vi "Vision Processing.vi"(4 "error in (no error)":errorcluster, 7 "Image Size":T1=enum."320x240") -> ()   [LabVIEW 2019]
doc: "This VI runs in parallel to other tasks. It gets images from the camera, processes them for color or shape and use that information to affect robot behavior."
uses:
  <vilib>/Rock Robotics/WPI/Camera/WPI_CameraImageSize.ctl
  <vilib>/Rock Robotics/WPI/Camera/WPI_CameraWhite Balance Values.ctl
  <vilib>/Rock Robotics/WPI/Camera/WPI_CameraExposure Values.ctl
  <vilib>/Rock Robotics/WPI/Camera/WPI_CameraFrameRate.ctl
  Robot Global Data.vi
  <vilib>/Rock Robotics/Network Tables/NT Write Number.vi
  <vilib>/Rock Robotics/Network Tables/NT Write Boolean.vi
  <vilib>/vision/driver/NI_Vision_Acquisition_Software.lvlib
  <vilib>/userDefined/High Color/IMAQdx.ctl
panel:
  out "x = y?":bool
  in  "Distance 2":u32
  out "f 2":dbl
  out "Object Size 2":u32
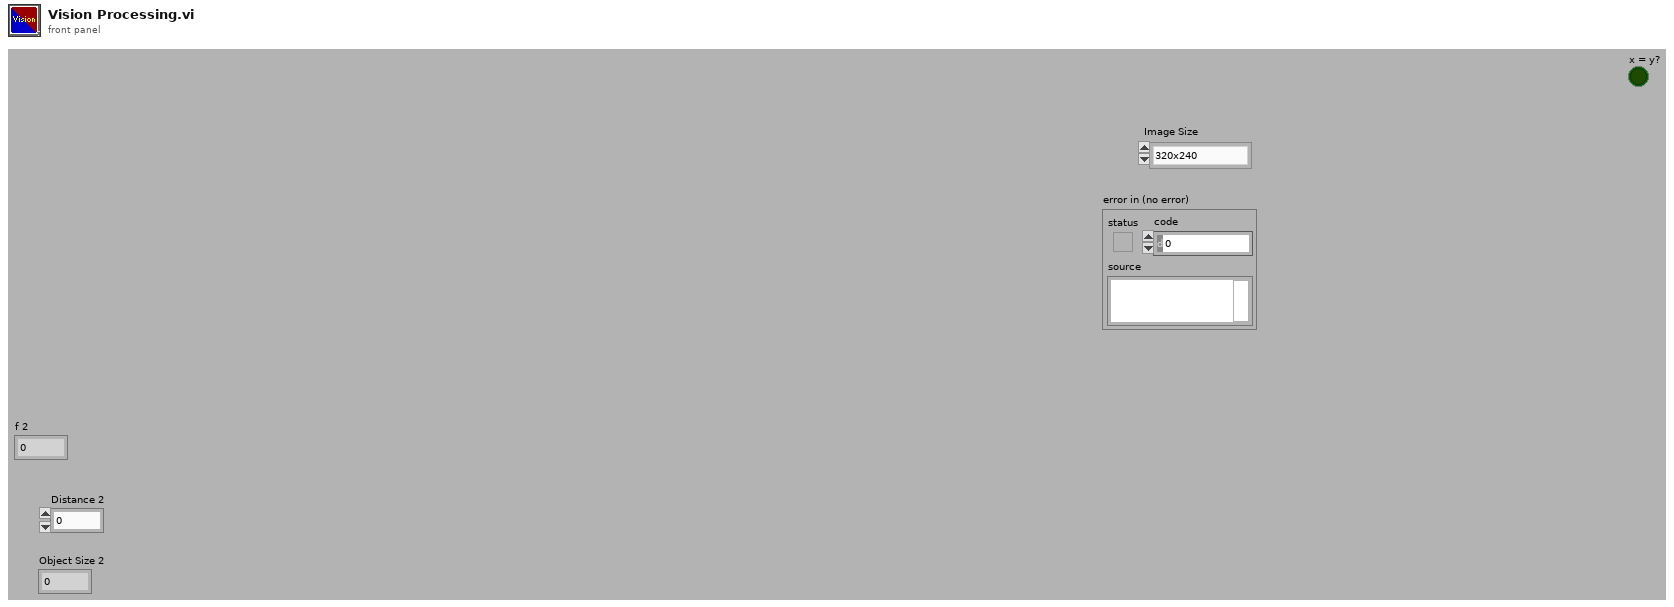
[diagram p1: front panel]
types:
  T1 = typedef "WPI_CameraImageSize.ctl" = enum16{"640x480", "320x240", "160x120", "Custom"}
  T2 = typedef "WPI_MotorControlDeviceRef.ctl" = cluster{"DeviceStatus":errorcluster, "Type":T3, "PWM":cluster{"PWM Channel":T4, "DeadBand":T5}, "CAN":cluster{"Device Number":u8, "SetOutput VI Ref":variant, "GetOutput VI Ref":variant, "Enable VI Ref":variant, "Disable VI Ref":variant, "Data":variant}, "Invert":bool, "DIO PWM":cluster{"PWM \"Enable\" Channel":T4, "DIOChannel":T6, "PWM Rate":dbl}}
  T3 = typedef "WPI_MotorControlType.ctl" = enum16{"PWM", "CAN", "DIO PWM"}
  T4 = typedef "FPGA_DIOPWMChannel.ctl" = enum8{"PWM 0", "PWM 1", "PWM 2", "PWM 3", "PWM 4", "PWM 5", "PWM 6", "PWM 7", "PWM 8", "PWM 9", "PWM MXP 0", "PWM MXP 1", "PWM MXP 2", "PWM MXP 3", "PWM MXP 4", "PWM MXP 5", "PWM MXP 6", "PWM MXP 7", "PWM MXP 8", "PWM MXP 9", "Invalid"}
  T5 = typedef "WPI_PWMDeadband.ctl" = cluster{"Name":string, "maxPositivePwm":i32, "minPositivePwm":i32, "centerPwm":i32, "maxNegativePwm":i32, "minNegativePwm":i32, "angularRange":u16}
  T6 = typedef "FPGA_DIOChannel.ctl" = enum8{"DIO 0", "DIO 1", "DIO 2", "DIO 3", "DIO 4", "DIO 5", "DIO 6", "DIO 7", "DIO 8", "DIO 9", "DIO MXP 0", "DIO MXP 1", "DIO MXP 2", "DIO MXP 3", "DIO MXP 4", "DIO MXP 5", "DIO MXP 6", "DIO MXP 7", "DIO MXP 8", "DIO MXP 9", "DIO MXP 10", "DIO MXP 11", "DIO MXP 12", "DIO MXP 13", "DIO MXP 14", "DIO MXP 15", "SPI Port CS1", "SPI Port CS2", "SPI Port CS3", "SPI Port MISO", "SPI Port MOSI", "Invalid"}
  T7 = typedef "WPI_CameraFrameRate.ctl" = u32
  T8 = typedef "WPI_CameraExposure Values.ctl" = enum16{"Auto", "Flicker-free 50 Hz", "Flicker-free 60 Hz", "Hold current", "Custom"}
  T9 = typedef "WPI_CameraWhite Balance Values.ctl" = enum16{"Auto", "Fixed indoor", "Fixed outdoor 1", "Fixed outdoor 2", "Fixed fluorescent 1", "Fixed fluorescent 2", "Hold current", "Custom"}
  T10 = typedef "IMAQdx.ctl" = refnum<k21>
  T11 = typedef "Image Type" = u32
  T12 = typedef "WPI_CameraDevRef.ctl" = cluster{"Camera Address":string, "CameraStatus":errorcluster}
  T13 = typedef "IMAQ Image.ctl" = refnum<image>
  T14 = cluster{"Global Rectangle":cluster{"x1Left":i32, "y1Top":i32, "x2Right":i32, "y2Bottom":i32}, "Centroid":cluster{"x":sgl, "y":sgl}, "Object Size":u32, "Score":dbl}[]
  T15 = cluster{"Global Rectangle":cluster{"x1Left":i32, "y1Top":i32, "x2Right":i32, "y2Bottom":i32}, "Centroid":cluster{"x":sgl, "y":sgl}, "Object Size":u32, "Score":dbl}
  T16 = cluster{"Shape Report[0]":cluster{"Global Rectangle":cluster{"x1Left":i32, "y1Top":i32, "x2Right":i32, "y2Bottom":i32}, "Centroid":cluster{"x":sgl, "y":sgl}, "Object Size":u32, "Score":dbl}, "Shape Report[1]":cluster{"Global Rectangle":cluster{"x1Left":i32, "y1Top":i32, "x2Right":i32, "y2Bottom":i32}, "Centroid":cluster{"x":sgl, "y":sgl}, "Object Size":u32, "Score":dbl}, "Shape Report[2]":cluster{"Global Rectangle":cluster{"x1Left":i32, "y1Top":i32, "x2Right":i32, "y2Bottom":i32}, "Centroid":cluster{"x":sgl, "y":sgl}, "Object Size":u32, "Score":dbl}, "Shape Report[3]":cluster{"Global Rectangle":cluster{"x1Left":i32, "y1Top":i32, "x2Right":i32, "y2Bottom":i32}, "Centroid":cluster{"x":sgl, "y":sgl}, "Object Size":u32, "Score":dbl}, "Shape Report[4]":cluster{"Global Rectangle":cluster{"x1Left":i32, "y1Top":i32, "x2Right":i32, "y2Bottom":i32}, "Centroid":cluster{"x":sgl, "y":sgl}, "Object Size":u32, "Score":dbl}, "Shape Report[5]":cluster{"Global Rectangle":cluster{"x1Left":i32, "y1Top":i32, "x2Right":i32, "y2Bottom":i32}, "Centroid":cluster{"x":sgl, "y":sgl}, "Object Size":u32, "Score":dbl}, "Shape Report[6]":cluster{"Global Rectangle":cluster{"x1Left":i32, "y1Top":i32, "x2Right":i32, "y2Bottom":i32}, "Centroid":cluster{"x":sgl, "y":sgl}, "Object Size":u32, "Score":dbl}, "Shape Report[7]":cluster{"Global Rectangle":cluster{"x1Left":i32, "y1Top":i32, "x2Right":i32, "y2Bottom":i32}, "Centroid":cluster{"x":sgl, "y":sgl}, "Object Size":u32, "Score":dbl}, "Shape Report[8]":cluster{"Global Rectangle":cluster{"x1Left":i32, "y1Top":i32, "x2Right":i32, "y2Bottom":i32}, "Centroid":cluster{"x":sgl, "y":sgl}, "Object Size":u32, "Score":dbl}}
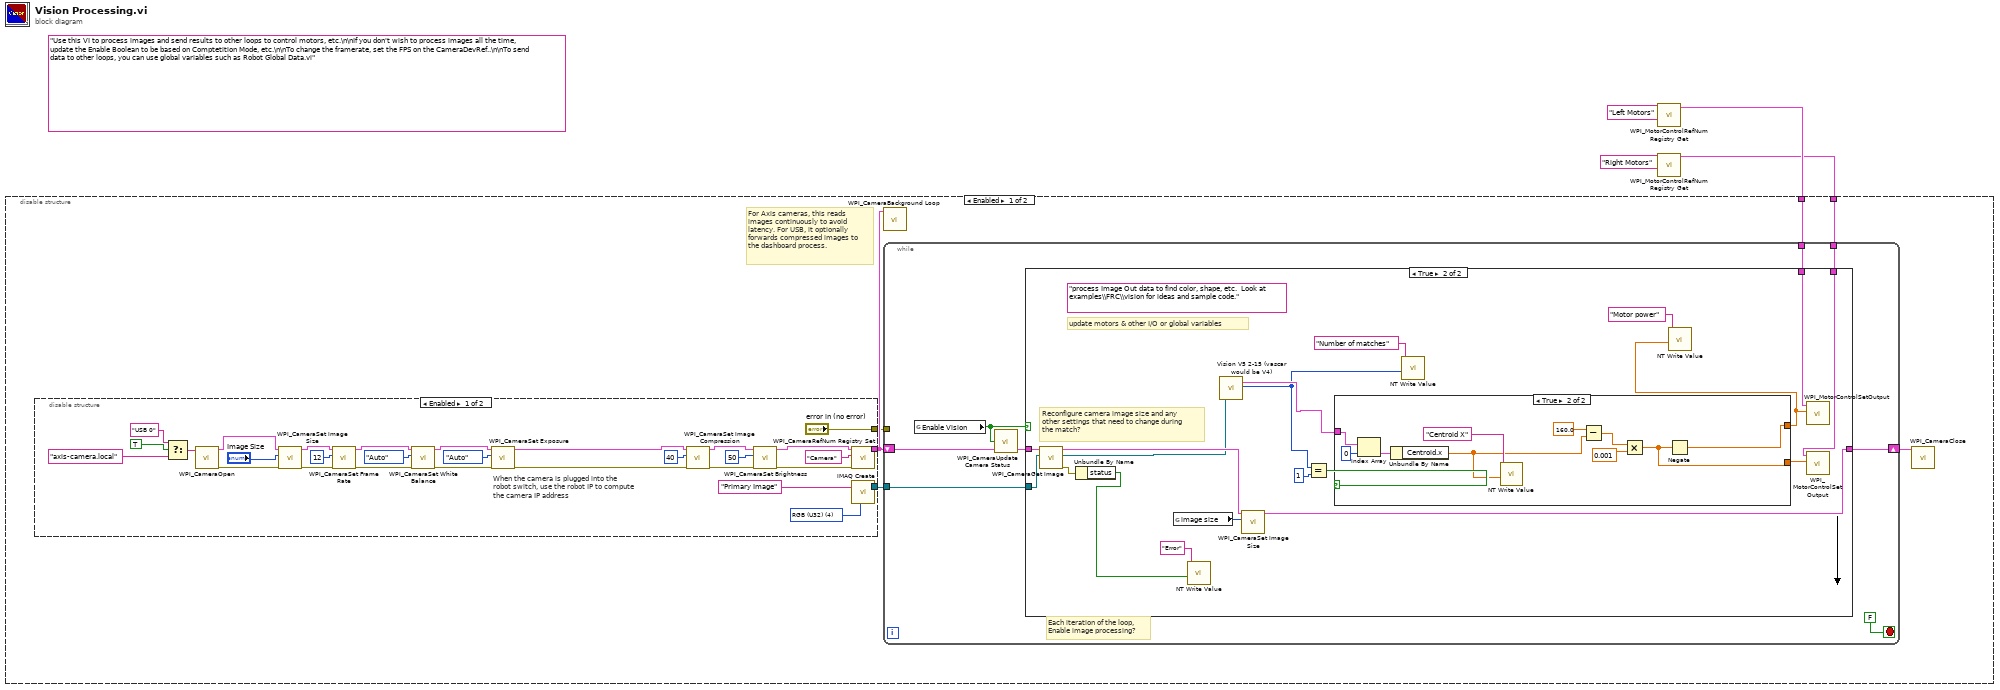
[diagram p0: block diagram]
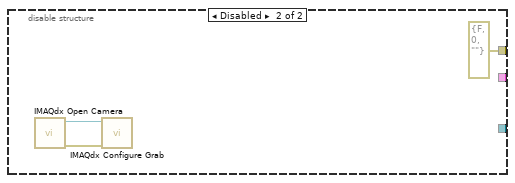
[diagram p2: hidden frame]
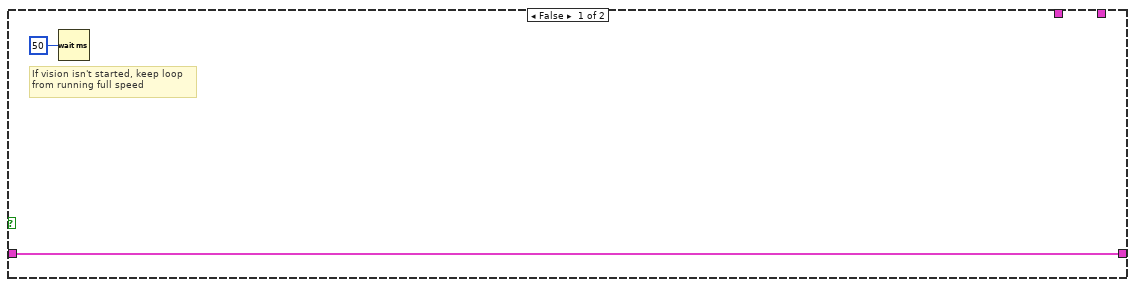
[diagram p3: hidden frame]
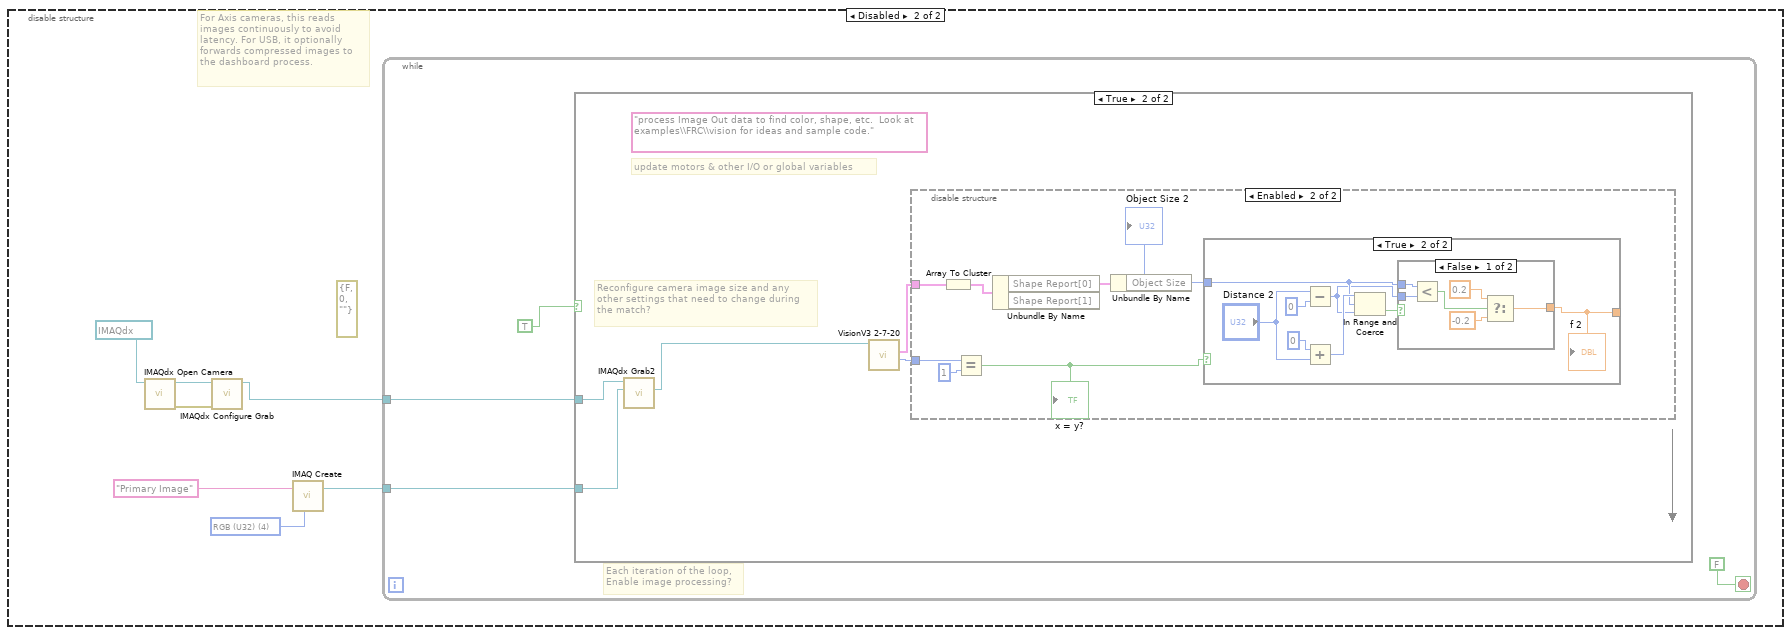
[diagram p5: hidden frame]
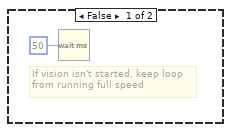
[diagram p6: hidden frame]
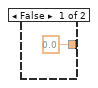
[diagram p8: hidden frame]
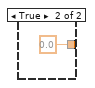
[diagram p9: hidden frame]
diagram:
  (unwired) "Use this VI to process images and send results to other loops to control motors, etc.\n\nIf you don't wish to process images all the time, update the Enable Boolean to be based on Comptetition Mode, etc.\n\nTo change the framerate, set the FPS on the CameraDevRef..\n\nTo send data to other loops, you can use global variables such as Robot Global Data.vi"
  n1 = call <vilib>:"WPI_MotorControlRefNum Registry Get.vi"("refnum name"="Left Motors") -> ("MotorControlDevRef"=w4:T2)  [unwired: 9 in, 1 out]
  n2 = call <vilib>:"WPI_MotorControlRefNum Registry Get.vi"("refnum name"="Right Motors") -> ("MotorControlDevRef"=w3:T2)  [unwired: 9 in, 1 out]
  n3 = disable-structure shown="Enabled" {
    disable-tunnel: w4 -> [w6 _]
    disable-tunnel: w3 -> [w5 _]
    frame Enabled {
      # "For Axis cameras, this reads\nimages continuously to avoid\nlatency. For USB, it optionally\nforwards compressed images to\nthe dashboard process."
      n4 = disable-structure shown="Enabled" {
        disable-tunnel: [w38 w41] -> w10
        disable-tunnel: [w17 _] -> w9
        disable-tunnel: ["error in (no error)" errorcluster {"status"=FALSE, "code"=0, "source"=""} ("error in (no error)")] -> w7
        frame Enabled {
          w40 = T11 4 items=["Grayscale (U8)", "Grayscale (I16)", "Grayscale (SGL)", "Complex (CSG)", "RGB (U32)", "HSL (U32)", "RGB (U64)"] ("Image Type")
          # "When the camera is plugged into the\nrobot switch, use the robot IP to compute\nthe camera IP address"
          n5 = Select(t="USB 0" ("format string"), s=TRUE ("dot notation? (F)"), f="axis-camera.local" ("format string")) -> (s? t:f=w12:string)
          n6 = call <vilib>:"WPI_CameraOpen.vi"("Camera Address"=w12) -> ("error out"=w28:errorcluster, "CameraDevRef"=w29:T12)  [unwired: 1 in, 8 out]
          n7 = call <vilib>:"WPI_CameraSet Image Size.vi"("error in (no error)"=w28, "Image Size"="Image Size", "CameraDevRef"=w29) -> ("error out"=w27:errorcluster, "CameraDevRef Out"=w30:T12)  [unwired: 1 in, 6 out]
          n8 = call <vilib>:"WPI_CameraSet Frame Rate.vi"("error in (no error)"=w27, "Frame Rate (fps)"=T7 12, "CameraDevRef"=w30) -> ("error out"=w26:errorcluster, "CameraDevRef Out"=w32:T12)  [unwired: 7 out]
          n9 = call <vilib>:"WPI_CameraSet White Balance.vi"("error in (no error)"=w26, "White Balance"=WPI_CameraWhite_Balance_Values."Auto", "CameraDevRef"=w32) -> ("error out"=w25:errorcluster, "CameraDevRef Out"=w31:T12)  [unwired: 1 in, 6 out]
          n10 = call <vilib>:"WPI_CameraSet Exposure.vi"("error in (no error)"=w25, "Exposure"=WPI_CameraExposure_Values."Auto", "CameraDevRef"=w31) -> ("error out"=w24:errorcluster, "CameraDevRef Out"=w34:T12)  [unwired: 1 in, 6 out]
          n11 = call <vilib>:"WPI_CameraSet Image Compression.vi"("error in (no error)"=w24, "Compression"=40, "CameraDevRef"=w34) -> ("error out"=w23:errorcluster, "CameraDevRef Out"=w33:T12)  [unwired: 7 out]
          n12 = call <vilib>:"WPI_CameraSet Brightness.vi"("error in (no error)"=w23, "Brightness"=50, "CameraDevRef"=w33) -> ("error out"=w21:errorcluster, "CameraDevRef Out"=w22:T12)  [unwired: 1 in, 6 out]
          n13 = call <vilib>:"WPI_CameraRefNum Registry Set.vi"("error in (no error)"=w21, "refnum name"="Camera", "CameraDevRef"=w22) -> ("CameraDevRef"=w17:T12)  [unwired: 1 in, 7 out]
          n14 = call "IMAQ Create"("Image Name"="Primary Image", "Image Type"=w40) -> ("New Image"=w38:T13)  [unwired: 2 in, 2 out]
        }
        frame Disabled {
          n15 = call <vilib>:"IMAQdx Open Camera.vi"() -> ("error out"=w45:errorcluster, "Session Out"=w43:T10)  [unwired: 10 in]
          n16 = call <vilib>:"IMAQdx Configure Grab.vi"("error in"=w45, "Session In"=w43) -> ("error out"=w46:errorcluster, "Session Out"=w44:T10)  [unwired: 8 in]
        }
      }
      n17 = call <vilib>:"WPI_CameraBackground Loop.vi"("CameraDevRef"=w9) -> ()  [unwired: 11 in]
      n18 = while {
        shift-right: [w53] -> w8
        shift-left: w9 -> [w51]
        tunnel: w10 -> [w52]
        tunnel: w7 -> [_]
        tunnel: w6 -> [w48]
        tunnel: w5 -> [w47]
        stop <- FALSE stop-if-true
        # "Each iteration of the loop,\nEnable image processing?"
        n19 = global read "Robot Global Data.vi" "Enable Vision"() -> (w49:bool)
        n20 = call <vilib>:"WPI_CameraUpdate Camera Status.vi"("CameraDevRef In"=w51, "Enable Vision"=w49) -> ("CameraDevRef Out"=w50:T12)  [unwired: 3 in]
        n21 = case shown="True" w49 {
          tunnel: w52 -> [_ w71]
          tunnel: [w56 w75] -> w53
          tunnel: w50 -> [w56 w73]
          tunnel: w48 -> [_ w60]
          tunnel: w47 -> [_ w59]
          frame False {
            # "If vision isn't started, keep loop\nfrom running full speed"
            n22 = Wait (ms)(milliseconds to wait=u32 50) -> ()  [unwired: 1 out]
          }
          frame True {
            (unwired) "process Image Out data to find color, shape, etc.  Look at examples\\FRC\\vision for ideas and sample code."
            # "update motors & other I/O or global variables"
            # "Reconfigure camera image size and any\nother settings that need to change during\nthe match?"
            n23 = call <vilib>:"WPI_CameraGet Image.vi"("Image"=w71, "CameraDevRef"=w73) -> ("error out"=w64:errorcluster, "Image Out"=w68:T13, "CameraDevRef Out"=w72:T12)  [unwired: 1 in, 6 out]
            n24 = Unbundle By Name(w64) -> ("status"=w62:bool)
            n25 = global read "Robot Global Data.vi" "image size"() -> (w74:T1)
            n26 = call-poly <vilib>:"NT Write Value.vi"("Boolean"=w62, "Name"="Error") -> ()  [unwired: 9 in, 1 out]
            n27 = call "Vision V5 2-15 (vascar would be V4).vi"("Image in"=w68) -> ("Shape Report (calibrated)"=w67:T14, "Number of Matches"=w65:i32)  [unwired: 15 in, 2 out]
            n28 = call <vilib>:"WPI_CameraSet Image Size.vi"("Image Size"=w74, "CameraDevRef"=w72) -> ("CameraDevRef Out"=w75:T12)  [unwired: 2 in, 7 out]
            n29 = Equal?(x=w65, y=1) -> (x = y?=w66:bool)
            n30 = case shown="True" w66 {
              tunnel: w67 -> [_ w85]
              tunnel: [_ w78] -> w58
              tunnel: [_ w77] -> w57
              frame False {
              }
              frame True {
                n31 = Index Array(array=w85, index=0) -> (element=w83:T15)
                n32 = Unbundle By Name(w83) -> ("Centroid.x"=w76:sgl)
                n33 = call-poly <vilib>:"NT Write Value.vi"("Numeric"=w76, "Name"="Centroid X") -> ()  [unwired: 9 in, 1 out]
                n34 = Subtract(x=160.0, y=w76) -> (x-y=w80:dbl)
                n35 = Multiply(x=w80, y=0.001) -> (x*y=w77:dbl)
                n36 = Negate(x=w77) -> (-x=w78:dbl)
              }
            }
            n37 = call-poly <vilib>:"NT Write Value.vi"("Numeric"=w65, "Name"="Number of matches") -> ()  [unwired: 9 in, 1 out]
            n38 = call-poly <vilib>:"NT Write Value.vi"("Numeric"=w58, "Name"="Motor power") -> ()  [unwired: 9 in, 1 out]
            n39 = call <vilib>:"WPI_MotorControlSetOutput.vi"("Output"=w58, "MotorControlDevRef"=w60) -> ()  [unwired: 7 in, 3 out]
            n40 = call <vilib>:"WPI_MotorControlSetOutput.vi"("Output"=w57, "MotorControlDevRef"=w59) -> ()  [unwired: 7 in, 3 out]
          }
        }
      }
      n41 = call <vilib>:"WPI_CameraClose.vi"("CameraDevRef"=w8) -> ()  [unwired: 1 in, 10 out]
    }
    frame Disabled {
      w89 = T11 4 items=["Grayscale (U8)", "Grayscale (I16)", "Grayscale (SGL)", "Complex (CSG)", "RGB (U32)", "HSL (U32)", "RGB (U64)"] ("Image Type")
      (unwired) errorcluster {"status"=FALSE, "code"=0, "source"=""} ("error in (no error)")
      # "For Axis cameras, this reads\nimages continuously to avoid\nlatency. For USB, it optionally\nforwards compressed images to\nthe dashboard process."
      n42 = call <vilib>:"IMAQdx Open Camera.vi"("Session In"=T10 "cam0") -> ("error out"=w92:errorcluster, "Session Out"=w91:T10)  [unwired: 9 in]
      n43 = call <vilib>:"IMAQdx Configure Grab.vi"("error in"=w92, "Session In"=w91) -> ("Session Out"=w90:T10)  [unwired: 8 in, 1 out]
      n44 = call "IMAQ Create"("Image Name"="Primary Image", "Image Type"=w89) -> ("New Image"=w87:T13)  [unwired: 2 in, 2 out]
      n45 = while {
        tunnel: w90 -> [w95]
        tunnel: w87 -> [w94]
        stop <- FALSE stop-if-true
        # "Each iteration of the loop,\nEnable image processing?"
        n46 = case shown="True" TRUE {
          tunnel: w95 -> [_ w100]
          tunnel: w94 -> [_ w98]
          frame False {
            # "If vision isn't started, keep loop\nfrom running full speed"
            n47 = Wait (ms)(milliseconds to wait=u32 50) -> ()  [unwired: 1 out]
          }
          frame True {
            (unwired) "process Image Out data to find color, shape, etc.  Look at examples\\FRC\\vision for ideas and sample code."
            # "update motors & other I/O or global variables"
            # "Reconfigure camera image size and any\nother settings that need to change during\nthe match?"
            n48 = call <vilib>:"IMAQdx Grab2.vi"("Image In"=w98, "Session In"=w100) -> ("Image Out"=w99:T13)  [unwired: 6 in, 3 out]
            n49 = call "VisionV3 2-7-20.vi"("Image In"=w99) -> ("Number of Matches"=w101:i32, "Shape Report"=w102:T14)  [unwired: 6 in, 2 out]
            n50 = disable-structure shown="Enabled" {
              disable-tunnel: w102 -> [_ w106]
              disable-tunnel: w101 -> [_ w109]
              frame Disabled {
                # "write globals"
                # "do something"
              }
              frame Enabled {
                n51 = Array To Cluster(array=w106) -> (cluster=w105:T16)
                n52 = Equal?(x=w109, y=1) -> (x = y?=w107:bool)
                "x = y?" <- w107
                n53 = Unbundle By Name(w105) -> ("Shape Report[0]"=w104:T15)  [unwired: 1 out]
                n54 = Unbundle By Name(w104) -> ("Object Size"=w103:u32)
                "Object Size 2" <- w103
                n55 = case shown="True" w107 {
                  tunnel: w103 -> [_ w113]
                  tunnel: [0.0 ("f") w111] -> _
                  frame False {
                  }
                  frame True {
                    n56 = Subtract(x="Distance 2", y=u32 0) -> (x-y=w112:u32)
                    n57 = Add(x=u32 0, y="Distance 2") -> (x+y=w118:u32)
                    n58 = In Range and Coerce(upper limit=w118, x=w113, lower limit=w112) -> (In Range?=w114:bool)  [unwired: 1 out]
                    n59 = case shown="False" w114 {
                      tunnel: [w119 0.0 ("f")] -> w111
                      tunnel: w113 -> [w124 _]
                      tunnel: w112 -> [w123 _]
                      frame False {
                        n60 = Less?(x=w124, y=w123) -> (x < y?=w122:bool)
                        n61 = Select(t=0.2, s=w122, f=-0.2) -> (s? t:f=w119:dbl)
                      }
                      frame True {
                      }
                    }
                    "f 2" <- w111
                  }
                }
              }
            }
          }
        }
      }
    }
  }
